vi "SetRawArray.vi"(0 "reference in":refnum<class "AI.lvclass">, 5 "RAW":dbl[](array[numeric]), 11 "error in (no error)":errorcluster) -> (4 "reference out":refnum<class "AI.lvclass">, 15 "error out":errorcluster)   [LabVIEW 2019, in "AI.lvclass"]
uses:
  AI.lvclass
  C:/Users/ANENKOV_V1/Desktop/src/Proccess_class/Proccess.lvclass
  AI.lvclass/AI.ctl
  PiecedLinearScale_class/Scale_PiecedLinear.lvclass/Scale_PiecedLinear.ctl
  Proccess_class/Proccess.lvclass/Proccess.ctl
  Logger_class/Logger.lvclass/Logger.ctl
  AnalogComparator_class/AnalogComparator.lvclass/AnalogComparator.ctl
  PiecedLinearScale_class/RawToScaled.vi
  subvis/Average.vi
  subvis/Loop Time Const.vi
  HandleRanges.vi
  HandleAlarms.vi
  private/WriteToDb.vi
  AnalogComparator_class/SetValue.vi
  Logger_class/Enqueue Signal.vi
  Proccess_class/GetNames.vi
  Proccess_class/GetLogger.vi
  <vilib>/gmath/interp.llb/Interpolate 1D.vi
  <vilib>/Utility/error.llb/Error Cluster From Error Code.vi
  AnalogComparator_class/SendToDb.vi
  <vilib>/Analysis/NI_AALBase.lvlib
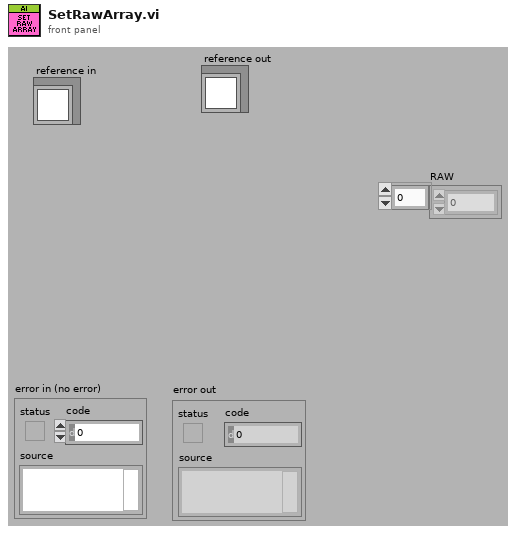
[diagram p1: front panel]
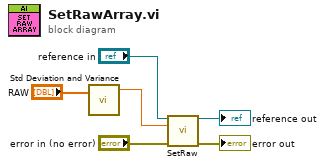
[diagram p0: block diagram]
diagram:
  n1 = call <vilib>:"Std Deviation and Variance.vi"("X"="RAW") -> ("mean"=w4:dbl)  [unwired: 1 in, 2 out]
  n2 = call "SetRaw.vi"("reference in"="reference in", "raw mean"=w4, "error in (no error)"="error in (no error)") -> ("reference out"=→"reference out":refnum<class "AI.lvclass">, "error out"=→"error out":errorcluster)  [unwired: 11 in]
